vi "Global_WC_Drive_Zero_Encoders.vi"() -> ()   [LabVIEW 2017]
panel:
  in  "Zero Encoders":bool
  # "The Names of the Data items in the Global Variable MUST describe who the Single Writer is\nNaming Convention of all Data Items is:   Lib Name_Loop Name (SM or SEN or ACT)_Data Name\nExample   Drive_ACT_X axis;  GameController_SEN_JoystickLeft;  Hopper_SM_AgitatorSpeed"
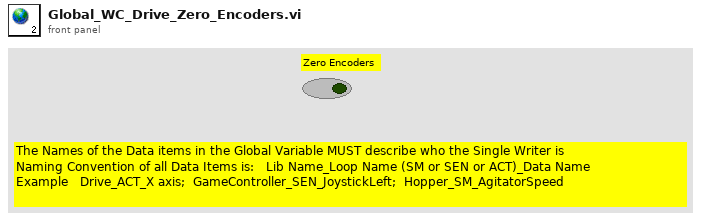
[diagram p1: front panel]
diagram:
